vi "main.vi"() -> ()   [LabVIEW 2023] (continued)
"ScaleFac"=0.1, "ScaleOff"=0.0}, {"1802D0A6", "Frame"="INVTEACStat2\ndatabase", "NameShort"="INVTEACStat2OUTVolt", "StartBit"=16, "NumBits"=16, "Min"=0.0, "Max"=1000.0, "ScaleFac"=0.1, "ScaleOff"=0.0}, {"1801D0A5", "Frame"="INVTEHPSStat\ndatabase", "NameShort"="INVTEHPSFaultLvl", "StartBit"=8, "NumBits"=2, "Min"=0.0, "Max"=3.0, "ScaleFac"=1.0, "ScaleOff"=0.0}, {"1801D0A5", "Frame"="INVTEHPSStat\ndatabase", "NameShort"="INVTEHPSStatErrCode", "StartBit"=0, "NumBits"=8, "Min"=0.0, "Max"=255.0, "ScaleFac"=1.0, "ScaleOff"=0.0}, {"1801D0A5", "Frame"="INVTEHPSStat\ndatabase", "NameShort"="INVTEHPSStatFaultStat", "StartBit"=14, "NumBits"=2, "Min"=0.0, "Max"=3.0, "ScaleFac"=1.0, "ScaleOff"=0.0}, {"1801D0A5", "Frame"="INVTEHPSStat\ndatabase", "NameShort"="INVTEHPSStatINVolt", "StartBit"=16, "NumBits"=16, "Min"=0.0, "Max"=1000.0, "ScaleFac"=0.1, "ScaleOff"=0.0}, {"1801D0A5", "Frame"="INVTEHPSStat\ndatabase", "NameShort"="INVTEHPSStatInvertorTemp", "StartBit"=48, "NumBits"=8, "Min"=-40.0, "Max"=150.0, "ScaleFac"=1.0, "ScaleOff"=-40.0}, {"1801D0A5", "Frame"="INVTEHPSStat\ndatabase", "NameShort"="INVTEHPSStatLife", "StartBit"=56, "NumBits"=8, "Min"=0.0, "Max"=255.0, "ScaleFac"=1.0, "ScaleOff"=0.0}, {"1801D0A5", "Frame"="INVTEHPSStat\ndatabase", "NameShort"="INVTEHPSStatMtrTemp", "StartBit"=32, "NumBits"=8, "Min"=-40.0, "Max"=200.0, "ScaleFac"=1.0, "ScaleOff"=-40.0}, {"1801D0A5", "Frame"="INVTEHPSStat\ndatabase", "NameShort"="INVTEHPSStatPowerStat", "StartBit"=10, "NumBits"=2, "Min"=0.0, "Max"=3.0, "ScaleFac"=1.0, "ScaleOff"=0.0}, {"1801D0A5", "Frame"="INVTEHPSStat\ndatabase", "NameShort"="INVTEHPSStatWorkStat", "StartBit"=12, "NumBits"=2, "Min"=0.0, "Max"=3.0, "ScaleFac"=1.0, "ScaleOff"=0.0}, {"1802D0A5", "Frame"="INVTEHPSStat2\ndatabase", "NameShort"="INVTEHPSStat2INCurr", "StartBit"=48, "NumBits"=16, "Min"=0.0, "Max"=6553.5, "ScaleFac"=0.1, "ScaleOff"=0.0}, {"1802D0A5", "Frame"="INVTEHPSStat2\ndatabase", "NameShort"="INVTEHPSStat2Mtrrpm", "StartBit"=0, "NumBits"=16, "Min"=-5000.0, "Max"=5000.0, "ScaleFac"=0.5, "ScaleOff"=-5000.0}, {"1802D0A5", "Frame"="INVTEHPSStat2\ndatabase", "NameShort"="INVTEHPSStat2OUTCurr", "StartBit"=32, "NumBits"=16, "Min"=0.0, "Max"=500.0, "ScaleFac"=0.1, "ScaleOff"=0.0}, {"1802D0A5", "Frame"="INVTEHPSStat2\ndatabase", "NameShort"="INVTEHPSStat2OUTVolt", "StartBit"=16, "NumBits"=16, "Min"=0.0, "Max"=1000.0, "ScaleFac"=0.1, "ScaleOff"=0.0}, {"1801D0D7", "Frame"="INVTInsulationTester\ndatabase", "NameShort"="INVTInsulationTestErrorLv", "StartBit"=32, "NumBits"=8, "Min"=0.0, "Max"=255.0, "ScaleFac"=1.0, "ScaleOff"=0.0}, {"1801D0D7", "Frame"="INVTInsulationTester\ndatabase", "NameShort"="INVTInsulationTestLife", "StartBit"=40, "NumBits"=8, "Min"=0.0, "Max"=255.0, "ScaleFac"=1.0, "ScaleOff"=0.0}, {"1801D0D7", "Frame"="INVTInsulationTester\ndatabase", "NameShort"="INVTInsulationTestNEGtoGNDResist", "StartBit"=16, "NumBits"=16, "Min"=0.0, "Max"=65535.0, "ScaleFac"=1.0, "ScaleOff"=0.0}, {"1801D0D7", "Frame"="INVTInsulationTester\ndatabase", "NameShort"="INVTInsulationTestPOStoGNDResist", "StartBit"=0, "NumBits"=16, "Min"=0.0, "Max"=65535.0, "ScaleFac"=1.0, "ScaleOff"=0.0}, {"1801D0D7", "Frame"="INVTInsulationTester\ndatabase", "NameShort"="INVTInsulationTestStat", "StartBit"=48, "NumBits"=8, "Min"=0.0, "Max"=255.0, "ScaleFac"=1.0, "ScaleOff"=0.0}, {"18F301A8", "Frame"="INVTPDU\ndatabase", "NameShort"="INVTPDUACHVLoopStat", "StartBit"=26, "NumBits"=2, "Min"=0.0, "Max"=3.0, "ScaleFac"=1.0, "ScaleOff"=0.0}, {"18F301A8", "Frame"="INVTPDU\ndatabase", "NameShort"="INVTPDUACPrechrgRlyStat", "StartBit"=20, "NumBits"=2, "Min"=0.0, "Max"=3.0, "ScaleFac"=1.0, "ScaleOff"=0.0}, {"18F301A8", "Frame"="INVTPDU\ndatabase", "NameShort"="INVTPDUACRlyStat", "StartBit"=22, "NumBits"=2, "Min"=0.0, "Max"=3.0, "ScaleFac"=1.0, "ScaleOff"=0.0}, {"18F301A8", "Frame"="INVTPDU\ndatabase", "NameShort"="INVTPDUFaultLvl", "StartBit"=32, "NumBits"=2, "Min"=0.0, "Max"=3.0, "ScaleFac"=1.0, "ScaleOff"=0.0}, {"18F301A8", "Frame"="INVTPDU\ndatabase", "NameShort"="INVTPDULife", "StartBit"=56, "NumBits"=8, "Min"=0.0, "Max"=255.0, "ScaleFac"=1.0, "ScaleOff"=0.0}, {"18F301A8", "Frame"="INVTPDU\ndatabase", "NameShort"="INVTPDUMCUHVLoopStat", "StartBit"=2, "NumBits"=2, "Min"=0.0, "Max"=3.0, "ScaleFac"=1.0, "ScaleOff"=0.0}, {"18F301A8", "Frame"="INVTPDU\ndatabase", "NameShort"="INVTPDUMCUMainRlyStat", "StartBit"=4, "NumBits"=2, "Min"=0.0, "Max"=3.0, "ScaleFac"=1.0, "ScaleOff"=0.0}, {"18F301A8", "Frame"="INVTPDU\ndatabase", "NameShort"="INVTPDUMCUPrechrgRlyStat", "StartBit"=6, "NumBits"=2, "Min"=0.0, "Max"=3.0, "ScaleFac"=1.0, "ScaleOff"=0.0}, {"18F301A8", "Frame"="INVTPDU\ndatabase", "NameShort"="INVTPDUStat", "StartBit"=0, "NumBits"=2, "Min"=0.0, "Max"=3.0, "ScaleFac"=1.0, "ScaleOff"=0.0}, {"18F301B8", "Frame"="INVTPDU2\ndatabase", "NameShort"="INVTPDU2INVolt", "StartBit"=0, "NumBits"=16, "Min"=0.0, "Max"=6553.5, "ScaleFac"=0.1, "ScaleOff"=0.0}, {"18F43A17", "Frame"="IP\ndatabase", "NameShort"="IP24V", "StartBit"=0, "NumBits"=8, "Min"=0.0, "Max"=50.0, "ScaleFac"=0.2, "ScaleOff"=0.0}, {"18F43A17", "Frame"="IP\ndatabase", "NameShort"="IPACCKeyPosnStat", "StartBit"=15, "NumBits"=1, "Min"=0.0, "Max"=1.0, "ScaleFac"=1.0, "ScaleOff"=0.0}, {"18F43A17", "Frame"="IP\ndatabase", "NameShort"="IPFrontAirReservoirPressure", "StartBit"=16, "NumBits"=8, "Min"=0.0, "Max"=1.0, "ScaleFac"=0.01, "ScaleOff"=0.0}, {"18F43A17", "Frame"="IP\ndatabase", "NameShort"="IPFrontDoorStat", "StartBit"=10, "NumBits"=1, "Min"=0.0, "Max"=1.0, "ScaleFac"=1.0, "ScaleOff"=0.0}, {"18F43A17", "Frame"="IP\ndatabase", "NameShort"="IPHandbrkStat", "StartBit"=12, "NumBits"=1, "Min"=0.0, "Max"=1.0, "ScaleFac"=1.0, "ScaleOff"=0.0}, {"18F43A17", "Frame"="IP\ndatabase", "NameShort"="IPHatchDoorStat", "StartBit"=11, "NumBits"=1, "Min"=0.0, "Max"=1.0, "ScaleFac"=1.0, "ScaleOff"=0.0}, {"18F43A17", "Frame"="IP\ndatabase", "NameShort"="IPLife", "StartBit"=56, "NumBits"=8, "Min"=0.0, "Max"=255.0, "ScaleFac"=1.0, "ScaleOff"=0.0}, {"18F43A17", "Frame"="IP\ndatabase", "NameShort"="IPMidDoorStat", "StartBit"=9, "NumBits"=1, "Min"=0.0, "Max"=1.0, "ScaleFac"=1.0, "ScaleOff"=0.0}, {"18F43A17", "Frame"="IP\ndatabase", "NameShort"="IPONKeyPosnStat", "StartBit"=14, "NumBits"=1, "Min"=0.0, "Max"=1.0, "ScaleFac"=1.0, "ScaleOff"=0.0}, {"18F43A17", "Frame"="IP\ndatabase", "NameShort"="IPRearAirReservoirPressure", "StartBit"=24, "NumBits"=8, "Min"=0.0, "Max"=1.0, "ScaleFac"=0.01, "ScaleOff"=0.0}, {"18F43A17", "Frame"="IP\ndatabase", "NameShort"="IPRearDoorStat", "StartBit"=8, "NumBits"=1, "Min"=0.0, "Max"=1.0, "ScaleFac"=1.0, "ScaleOff"=0.0}, {"18F43A17", "Frame"="IP\ndatabase", "NameShort"="IPSmokeDetectStat", "StartBit"=13, "NumBits"=1, "Min"=0.0, "Max"=1.0, "ScaleFac"=1.0, "ScaleOff"=0.0}, {"18F43A17", "Frame"="IP\ndatabase", "NameShort"="IPSpeedLimitReq", "StartBit"=33, "NumBits"=1, "Min"=0.0, "Max"=1.0, "ScaleFac"=1.0, "ScaleOff"=0.0}, {"18F43A17", "Frame"="IP\ndatabase", "NameShort"="IPThrottleInterlockReq", "StartBit"=32, "NumBits"=1, "Min"=0.0, "Max"=1.0, "ScaleFac"=1.0, "ScaleOff"=0.0}, {"18A70017", "Frame"="IP2\ndatabase", "NameShort"="IP2ABSStat", "StartBit"=42, "NumBits"=2, "Min"=0.0, "Max"=3.0, "ScaleFac"=1.0, "ScaleOff"=0.0}, {"18A70017", "Frame"="IP2\ndatabase", "NameShort"="IP2AirConStat", "StartBit"=14, "NumBits"=2, "Min"=0.0, "Max"=3.0, "ScaleFac"=1.0, "ScaleOff"=0.0}, {"18A70017", "Frame"="IP2\ndatabase", "NameShort"="IP2AirFilterClogWarn", "StartBit"=10, "NumBits"=2, "Min"=0.0, "Max"=3.0, "ScaleFac"=1.0, "ScaleOff"=0.0}, {"18A70017", "Frame"="IP2\ndatabase", "NameShort"="IP2BrkPadsWornOutWarn", "StartBit"=8, "NumBits"=2, "Min"=0.0, "Max"=3.0, "ScaleFac"=1.0, "ScaleOff"=0.0}, {"18A70017", "Frame"="IP2\ndatabase", "NameShort"="IP2BrkPressureWarn", "StartBit"=2, "NumBits"=2, "Min"=0.0, "Max"=3.0, "ScaleFac"=1.0, "ScaleOff"=0.0}, {"18A70017", "Frame"="IP2\ndatabase", "NameShort"="IP2BrkStat", "StartBit"=36, "NumBits"=2, "Min"=0.0, "Max"=3.0, "ScaleFac"=1.0, "ScaleOff"=0.0}, {"18A70017", "Frame"="IP2\ndatabase", "NameShort"="IP2EHPSWarn", "StartBit"=4, "NumBits"=2, "Min"=0.0, "Max"=3.0, "ScaleFac"=1.0, "ScaleOff"=0.0}, {"18A70017", "Frame"="IP2\ndatabase", "NameShort"="IP2EngineOilTempWarn", "StartBit"=54, "NumBits"=2, "Min"=0.0, "Max"=3.0, "ScaleFac"=1.0, "ScaleOff"=0.0}, {"18A70017", "Frame"="IP2\ndatabase", "NameShort"="IP2FogLightSig", "StartBit"=26, "NumBits"=2, "Min"=0.0, "Max"=3.0, "ScaleFac"=1.0, "ScaleOff"=0.0}, {"18A70017", "Frame"="IP2\ndatabase", "NameShort"="IP2FrontDoorSig", "StartBit"=20, "NumBits"=2, "Min"=0.0, "Max"=3.0, "ScaleFac"=1.0, "ScaleOff"=0.0}, {"18A70017", "Frame"="IP2\ndatabase", "NameShort"="IP2FuelClogWarn", "StartBit"=52, "NumBits"=2, "Min"=0.0, "Max"=3.0, "ScaleFac"=1.0, "ScaleOff"=0.0}, {"18A70017", "Frame"="IP2\ndatabase", "NameShort"="IP2FuelGauge", "StartBit"=56, "NumBits"=8, "Min"=0.0, "Max"=100.0, "ScaleFac"=0.4, "ScaleOff"=0.0}, {"18A70017", "Frame"="IP2\ndatabase", "NameShort"="IP2FuelWarn", "StartBit"=12, "NumBits"=2, "Min"=0.0, "Max"=3.0, "ScaleFac"=1.0, "ScaleOff"=0.0}, {"18A70017", "Frame"="IP2\ndatabase", "NameShort"="IP2GearNSig", "StartBit"=16, "NumBits"=2, "Min"=0.0, "Max"=3.0, "ScaleFac"=1.0, "ScaleOff"=0.0}, {"18A70017", "Frame"="IP2\ndatabase", "NameShort"="IP2GearRSig", "StartBit"=18, "NumBits"=2, "Min"=0.0, "Max"=3.0, "ScaleFac"=1.0, "ScaleOff"=0.0}, {"18A70017", "Frame"="IP2\ndatabase", "NameShort"="IP2HandBrkStat", "StartBit"=38, "NumBits"=2, "Min"=0.0, "Max"=3.0, "ScaleFac"=1.0, "ScaleOff"=0.0}, {"18A70017", "Frame"="IP2\ndatabase", "NameShort"="IP2HeaterStat", "StartBit"=44, "NumBits"=2, "Min"=0.0, "Max"=3.0, "ScaleFac"=1.0, "ScaleOff"=0.0}, {"18A70017", "Frame"="IP2\ndatabase", "NameShort"="IP2HighBeamSig", "StartBit"=30, "NumBits"=2, "Min"=0.0, "Max"=3.0, "ScaleFac"=1.0, "ScaleOff"=0.0}, {"18A70017", "Frame"="IP2\ndatabase", "NameShort"="IP2HornSig", "StartBit"=24, "NumBits"=2, "Min"=0.0, "Max"=0.0, "ScaleFac"=1.0, "ScaleOff"=0.0}, {"18A70017", "Frame"="IP2\ndatabase", "NameShort"="IP2LeftTurnSig", "StartBit"=32, "NumBits"=2, "Min"=0.0, "Max"=3.0, "ScaleFac"=1.0, "ScaleOff"=0.0}, {"18A70017", "Frame"="IP2\ndatabase", "NameShort"="IP2LowBeamSig", "StartBit"=28, "NumBits"=2, "Min"=0.0, "Max"=3.0, "ScaleFac"=1.0, "ScaleOff"=0.0}, {"18A70017", "Frame"="IP2\ndatabase", "NameShort"="IP2LowWaterLvlWarn", "StartBit"=6, "NumBits"=2, "Min"=0.0, "Max"=3.0, "ScaleFac"=1.0, "ScaleOff"=0.0}, {"18A70017", "Frame"="IP2\ndatabase", "NameShort"="IP2MidDoorSig", "StartBit"=22, "NumBits"=2, "Min"=0.0, "Max"=3.0, "ScaleFac"=1.0, "ScaleOff"=0.0}, {"18A70017", "Frame"="IP2\ndatabase", "NameShort"="IP2OilFilterClogWarn", "StartBit"=50, "NumBits"=2, "Min"=0.0, "Max"=3.0, "ScaleFac"=1.0, "ScaleOff"=0.0}, {"18A70017", "Frame"="IP2\ndatabase", "NameShort"="IP2RegenLeverStat", "StartBit"=40, "NumBits"=2, "Min"=0.0, "Max"=3.0, "ScaleFac"=1.0, "ScaleOff"=0.0}, {"18A70017", "Frame"="IP2\ndatabase", "NameShort"="IP2RegenOverheatWarn", "StartBit"=46, "NumBits"=2, "Min"=0.0, "Max"=3.0, "ScaleFac"=1.0, "ScaleOff"=0.0}, {"18A70017", "Frame"="IP2\ndatabase", "NameShort"="IP2RightTurnSig", "StartBit"=34, "NumBits"=2, "Min"=0.0, "Max"=3.0, "ScaleFac"=1.0, "ScaleOff"=0.0}, {"18A70017", "Frame"="IP2\ndatabase", "NameShort"="IP2SmokeDetectorWarn", "StartBit"=48, "NumBits"=2, "Min"=0.0, "Max"=3.0, "ScaleFac"=1.0, "ScaleOff"=0.0}, {"18A70017", "Frame"="IP2\ndatabase", "NameShort"="IP2ThrottleInterlockWarn", "StartBit"=0, "NumBits"=2, "Min"=0.0, "Max"=3.0, "ScaleFac"=1.0, "ScaleOff"=0.0}, {"18FEC117", "Frame"="IPMileage\ndatabase", "NameShort"="IPMileageTotalOdometer", "StartBit"=0, "NumBits"=32, "Min"=0.0, "Max"=21055406.0, "ScaleFac"=0.005, "ScaleOff"=0.0}, {"18FEC117", "Frame"="IPMileage\ndatabase", "NameShort"="IPMileageTripA", "StartBit"=32, "NumBits"=32, "Min"=0.0, "Max"=21055406.0, "ScaleFac"=0.005, "ScaleOff"=0.0}, {"18F746E6", "Frame"="InsulationTesterS\ndatabase", "NameShort"="InsulatTesterSDetailedErrCode", "StartBit"=40, "NumBits"=8, "Min"=0.0, "Max"=255.0, "ScaleFac"=1.0, "ScaleOff"=0.0}, {"18F746E6", "Frame"="InsulationTesterS\ndatabase", "NameShort"="InsulatTesterSDeviceFailure", "StartBit"=53, "NumBits"=1, "Min"=0.0, "Max"=1.0, "ScaleFac"=1.0, "ScaleOff"=0.0}, {"18F746E6", "Frame"="InsulationTesterS\ndatabase", "NameShort"="InsulatTesterSHVLeakAlertLv", "StartBit"=0, "NumBits"=3, "Min"=0.0, "Max"=7.0, "ScaleFac"=1.0, "ScaleOff"=0.0}, {"18F746E6", "Frame"="InsulationTesterS\ndatabase", "NameShort"="InsulatTesterSHVNegInsultErr", "StartBit"=51, "NumBits"=1, "Min"=0.0, "Max"=1.0, "ScaleFac"=1.0, "ScaleOff"=0.0}, {"18F746E6", "Frame"="InsulationTesterS\ndatabase", "NameShort"="InsulatTesterSHVPosInsltErr", "StartBit"=50, "NumBits"=1, "Min"=0.0, "Max"=1.0, "ScaleFac"=1.0, "ScaleOff"=0.0}, {"18F746E6", "Frame"="InsulationTesterS\ndatabase", "NameShort"="InsulatTesterSLife", "StartBit"=56, "NumBits"=8, "Min"=0.0, "Max"=255.0, "ScaleFac"=1.0, "ScaleOff"=0.0}, {"18F746E6", "Frame"="InsulationTesterS\ndatabase", "NameShort"="InsulatTesterSLv1Alert", "StartBit"=48, "NumBits"=1, "Min"=0.0, "Max"=1.0, "ScaleFac"=1.0, "ScaleOff"=0.0}, {"18F746E6", "Frame"="InsulationTesterS\ndatabase", "NameShort"="InsulatTesterSLv2Alert", "StartBit"=49, "NumBits"=1, "Min"=0.0, "Max"=1.0, "ScaleFac"=1.0, "ScaleOff"=0.0}, {"18F746E6", "Frame"="InsulationTesterS\ndatabase", "NameShort"="InsulatTesterSNegInsulatResist", "StartBit"=24, "NumBits"=16, "Min"=0.0, "Max"=65535.0, "ScaleFac"=1.0, "ScaleOff"=0.0}, {"18F746E6", "Frame"="InsulationTesterS\ndatabase", "NameShort"="InsulatTesterSPosInsulatResist", "StartBit"=8, "NumBits"=16, "Min"=0.0, "Max"=65535.0, "ScaleFac"=1.0, "ScaleOff"=0.0}, {"18F746E6", "Frame"="InsulationTesterS\ndatabase", "NameShort"="InsulatTesterSWiringFailure", "StartBit"=52, "NumBits"=1, "Min"=0.0, "Max"=1.0, "ScaleFac"=1.0, "ScaleOff"=0.0}, {"18F11FF0", "Frame"="MCU1ElectricalStat\ndatabase", "NameShort"="MCU1CANBusConnectStat", "StartBit"=52, "NumBits"=1, "Min"=0.0, "Max"=1.0, "ScaleFac"=1.0, "ScaleOff"=0.0}, {"18F11FF0", "Frame"="MCU1ElectricalStat\ndatabase", "NameShort"="MCU1HPINCurr", "StartBit"=16, "NumBits"=16, "Min"=-1000.0, "Max"=1000.0, "ScaleFac"=0.1, "ScaleOff"=-1000.0}, {"18F11FF0", "Frame"="MCU1ElectricalStat\ndatabase", "NameShort"="MCU1HPINOvercurrErr", "StartBit"=43, "NumBits"=1, "Min"=0.0, "Max"=1.0, "ScaleFac"=1.0, "ScaleOff"=0.0}, {"18F11FF0", "Frame"="MCU1ElectricalStat\ndatabase", "NameShort"="MCU1HPINOvervoltErr", "StartBit"=40, "NumBits"=1, "Min"=0.0, "Max"=1.0, "ScaleFac"=1.0, "ScaleOff"=0.0}, {"18F11FF0", "Frame"="MCU1ElectricalStat\ndatabase", "NameShort"="MCU1HPINUndervoltErr", "StartBit"=44, "NumBits"=1, "Min"=0.0, "Max"=1.0, "ScaleFac"=1.0, "ScaleOff"=0.0}, {"18F11FF0", "Frame"="MCU1ElectricalStat\ndatabase", "NameShort"="MCU1HPINVolt", "StartBit"=0, "NumBits"=16, "Min"=0.0, "Max"=1000.0, "ScaleFac"=0.1, "ScaleOff"=0.0}, {"18F11FF0", "Frame"="MCU1ElectricalStat\ndatabase", "NameShort"="MCU1HVBattConnectStat", "StartBit"=55, "NumBits"=1, "Min"=0.0, "Max"=1.0, "ScaleFac"=1.0, "ScaleOff"=0.0}, {"18F11FF0", "Frame"="MCU1ElectricalStat\ndatabase", "NameShort"="MCU1HillStartStat", "StartBit"=39, "NumBits"=1, "Min"=0.0, "Max"=1.0, "ScaleFac"=1.0, "ScaleOff"=0.0}, {"18F11FF0", "Frame"="MCU1ElectricalStat\ndatabase", "NameShort"="MCU1KeyIgniteStat", "StartBit"=54, "NumBits"=1, "Min"=0.0, "Max"=1.0, "ScaleFac"=1.0, "ScaleOff"=0.0}, {"18F11FF0", "Frame"="MCU1ElectricalStat\ndatabase", "NameShort"="MCU1LVDCPowErr", "StartBit"=53, "NumBits"=1, "Min"=0.0, "Max"=1.0, "ScaleFac"=1.0, "ScaleOff"=0.0}, {"18F11FF0", "Frame"="MCU1ElectricalStat\ndatabase", "NameShort"="MCU1Life", "StartBit"=60, "NumBits"=4, "Min"=0.0, "Max"=15.0, "ScaleFac"=1.0, "ScaleOff"=0.0}, {"18F11FF0", "Frame"="MCU1ElectricalStat\ndatabase", "NameShort"="MCU1MCUErr", "StartBit"=33, "NumBits"=1, "Min"=0.0, "Max"=1.0, "ScaleFac"=1.0, "ScaleOff"=0.0}, {"18F11FF0", "Frame"="MCU1ElectricalStat\ndatabase", "NameShort"="MCU1McuOverheatErr", "StartBit"=46, "NumBits"=1, "Min"=0.0, "Max"=1.0, "ScaleFac"=1.0, "ScaleOff"=0.0}, {"18F11FF0", "Frame"="MCU1ElectricalStat\ndatabase", "NameShort"="MCU1McuTempAlert", "StartBit"=51, "NumBits"=1, "Min"=0.0, "Max"=1.0, "ScaleFac"=1.0, "ScaleOff"=0.0}, {"18F11FF0", "Frame"="MCU1ElectricalStat\ndatabase", "NameShort"="MCU1Mode", "StartBit"=34, "NumBits"=5, "Min"=0.0, "Max"=31.0, "ScaleFac"=1.0, "ScaleOff"=0.0}, {"18F11FF0", "Frame"="MCU1ElectricalStat\ndatabase", "NameShort"="MCU1MtrOverheatErr", "StartBit"=45, "NumBits"=1, "Min"=0.0, "Max"=1.0, "ScaleFac"=1.0, "ScaleOff"=0.0}, {"18F11FF0", "Frame"="MCU1ElectricalStat\ndatabase", "NameShort"="MCU1MtrOverspdErr", "StartBit"=47, "NumBits"=1, "Min"=0.0, "Max"=1.0, "ScaleFac"=1.0, "ScaleOff"=0.0}, {"18F11FF0", "Frame"="MCU1ElectricalStat\ndatabase", "NameShort"="MCU1MtrPosnSensorErr", "StartBit"=42, "NumBits"=1, "Min"=0.0, "Max"=1.0, "ScaleFac"=1.0, "ScaleOff"=0.0}, {"18F11FF0", "Frame"="MCU1ElectricalStat\ndatabase", "NameShort"="MCU1MtrTempAlert", "StartBit"=50, "NumBits"=1, "Min"=0.0, "Max"=1.0, "ScaleFac"=1.0, "ScaleOff"=0.0}, {"18F11FF0", "Frame"="MCU1ElectricalStat\ndatabase", "NameShort"="MCU1NoPermsToOp", "StartBit"=57, "NumBits"=1, "Min"=0.0, "Max"=1.0, "ScaleFac"=1.0, "ScaleOff"=0.0}, {"18F11FF0", "Frame"="MCU1ElectricalStat\ndatabase", "NameShort"="MCU1PermsToOp", "StartBit"=56, "NumBits"=1, "Min"=0.0, "Max"=1.0, "ScaleFac"=1.0, "ScaleOff"=0.0}, {"18F11FF0", "Frame"="MCU1ElectricalStat\ndatabase", "NameShort"="MCU1PhaseCurrErr", "StartBit"=32, "NumBits"=1, "Min"=0.0, "Max"=1.0, "ScaleFac"=1.0, "ScaleOff"=0.0}, {"18F11FF0", "Frame"="MCU1ElectricalStat\ndatabase", "NameShort"="MCU1PhaseUOvercurrErr", "StartBit"=48, "NumBits"=1, "Min"=0.0, "Max"=1.0, "ScaleFac"=1.0, "ScaleOff"=0.0}, {"18F11FF0", "Frame"="MCU1ElectricalStat\ndatabase", "NameShort"="MCU1PhaseWOvercurrErr", "StartBit"=49, "NumBits"=1, "Min"=0.0, "Max"=1.0, "ScaleFac"=1.0, "ScaleOff"=0.0}, {"18F120F0", "Frame"="MCU2MtrStat\ndatabase", "NameShort"="MCU2CurrentMtrRPM", "StartBit"=16, "NumBits"=16, "Min"=-12000.0, "Max"=12000.0, "ScaleFac"=1.0, "ScaleOff"=-12000.0}, {"18F120F0", "Frame"="MCU2MtrStat\ndatabase", "NameShort"="MCU2McuTemp", "StartBit"=56, "NumBits"=8, "Min"=-40.0, "Max"=210.0, "ScaleFac"=1.0, "ScaleOff"=-40.0}, {"18F120F0", "Frame"="MCU2MtrStat\ndatabase", "NameShort"="MCU2MtrActualTorq", "StartBit"=32, "NumBits"=16, "Min"=-3000.0, "Max"=3000.0, "ScaleFac"=0.1, "ScaleOff"=-3000.0}, {"18F120F0", "Frame"="MCU2MtrStat\ndatabase", "NameShort"="MCU2MtrPeakTorq", "StartBit"=0, "NumBits"=16, "Min"=-3000.0, "Max"=3000.0, "ScaleFac"=0.1, "ScaleOff"=-3000.0}, {"18F120F0", "Frame"="MCU2MtrStat\ndatabase", "NameShort"="MCU2MtrTemp", "StartBit"=48, "NumBits"=8, "Min"=-40.0, "Max"=210.0, "ScaleFac"=1.0, "ScaleOff"=-40.0}, {"18F121F0", "Frame"="MCU3ErrorStat\ndatabase", "NameShort"="MCU3DriveshaftTorq", "StartBit"=48, "NumBits"=16, "Min"=-3000.0, "Max"=3000.0, "ScaleFac"=0.1, "ScaleOff"=-3000.0}, {"18F121F0", "Frame"="MCU3ErrorStat\ndatabase", "NameShort"="MCU3ErrCode", "StartBit"=8, "NumBits"=8, "Min"=0.0, "Max"=255.0, "ScaleFac"=1.0, "ScaleOff"=0.0}, {"18F121F0", "Frame"="MCU3ErrorStat\ndatabase", "NameShort"="MCU3ErrLv", "StartBit"=4, "NumBits"=4, "Min"=0.0, "Max"=4.0, "ScaleFac"=1.0, "ScaleOff"=0.0}, {"18F121F0", "Frame"="MCU3ErrorStat\ndatabase", "NameShort"="MCU3HwVer", "StartBit"=27, "NumBits"=5, "Min"=0.0, "Max"=31.0, "ScaleFac"=1.0, "ScaleOff"=0.0}, {"18F121F0", "Frame"="MCU3ErrorStat\ndatabase", "NameShort"="MCU3SwVer", "StartBit"=16, "NumBits"=11, "Min"=0.0, "Max"=2047.0, "ScaleFac"=1.0, "ScaleOff"=0.0}, {"18F121F0", "Frame"="MCU3ErrorStat\ndatabase", "NameShort"="MCU3SysStat", "StartBit"=0, "NumBits"=4, "Min"=0.0, "Max"=6.0, "ScaleFac"=1.0, "ScaleOff"=0.0}, {"1FFFFFFC", "Frame"="PCINPUT\ndatabase", "NameShort"="PCRXMsg1", "StartBit"=0, "NumBits"=16, "Min"=0.0, "Max"=65.535, "ScaleFac"=0.001, "ScaleOff"=0.0}, {"1FFFFFFC", "Frame"="PCINPUT\ndatabase", "NameShort"="PCRXMsg3", "StartBit"=16, "NumBits"=16, "Min"=0.0, "Max"=65.535, "ScaleFac"=0.001, "ScaleOff"=0.0}, {"1FFFFFFC", "Frame"="PCINPUT\ndatabase", "NameShort"="PCRXMsg5", "StartBit"=32, "NumBits"=16, "Min"=0.0, "Max"=65.535, "ScaleFac"=0.001, "ScaleOff"=0.0}, {"1FFFFFFC", "Frame"="PCINPUT\ndatabase", "NameShort"="PCRXMsg7", "StartBit"=48, "NumBits"=16, "Min"=0.0, "Max"=65.535, "ScaleFac"=0.001, "ScaleOff"=0.0}, {"1FFFFFFD", "Frame"="PCOUTPUT\ndatabase", "NameShort"="PCTXMsg1", "StartBit"=0, "NumBits"=16, "Min"=0.0, "Max"=65.535, "ScaleFac"=0.001, "ScaleOff"=0.0}, {"1FFFFFFD", "Frame"="PCOUTPUT\ndatabase", "NameShort"="PCTXMsg3", "StartBit"=16, "NumBits"=16, "Min"=0.0, "Max"=65.535, "ScaleFac"=0.001, "ScaleOff"=0.0}, {"1FFFFFFD", "Frame"="PCOUTPUT\ndatabase", "NameShort"="PCTXMsg5", "StartBit"=32, "NumBits"=16, "Min"=0.0, "Max"=65.535, "ScaleFac"=0.001, "ScaleOff"=0.0}, {"1FFFFFFD", "Frame"="PCOUTPUT\ndatabase", "NameShort"="PCTXMsg7", "StartBit"=48, "NumBits"=16, "Min"=0.0, "Max"=65.535, "ScaleFac"=0.001, "ScaleOff"=0.0}, {"1FFFFFFE", "Frame"="PCRX\ndatabase", "NameShort"="PCRXMsg1", "StartBit"=0, "NumBits"=8, "Min"=0.0, "Max"=255.0, "ScaleFac"=1.0, "ScaleOff"=0.0}, {"1FFFFFFE", "Frame"="PCRX\ndatabase", "NameShort"="PCRXMsg2", "StartBit"=8, "NumBits"=8, "Min"=0.0, "Max"=255.0, "ScaleFac"=1.0, "ScaleOff"=0.0}, {"1FFFFFFE", "Frame"="PCRX\ndatabase", "NameShort"="PCRXMsg3", "StartBit"=16, "NumBits"=8, "Min"=0.0, "Max"=255.0, "ScaleFac"=1.0, "ScaleOff"=0.0}, {"1FFFFFFE", "Frame"="PCRX\ndatabase", "NameShort"="PCRXMsg4", "StartBit"=24, "NumBits"=8, "Min"=0.0, "Max"=255.0, "ScaleFac"=1.0, "ScaleOff"=0.0}, {"1FFFFFFE", "Frame"="PCRX\ndatabase", "NameShort"="PCRXMsg5", "StartBit"=32, "NumBits"=8, "Min"=0.0, "Max"=255.0, "ScaleFac"=1.0, "ScaleOff"=0.0}, {"1FFFFFFE", "Frame"="PCRX\ndatabase", "NameShort"="PCRXMsg6", "StartBit"=40, "NumBits"=8, "Min"=0.0, "Max"=255.0, "ScaleFac"=1.0, "ScaleOff"=0.0}, {"1FFFFFFE", "Frame"="PCRX\ndatabase", "NameShort"="PCRXMsg7", "StartBit"=48, "NumBits"=8, "Min"=0.0, "Max"=255.0, "ScaleFac"=1.0, "ScaleOff"=0.0}, {"1FFFFFFE", "Frame"="PCRX\ndatabase", "NameShort"="PCRXMsg8", "StartBit"=56, "NumBits"=8, "Min"=0.0, "Max"=255.0, "ScaleFac"=1.0, "ScaleOff"=0.0}, {"1FFFFFFF", "Frame"="PCTX\ndatabase", "NameShort"="PCTXMSDI_Gear", "StartBit"=0, "NumBits"=8, "Min"=0.0, "Max"=255.0, "ScaleFac"=1.0, "ScaleOff"=0.0}, {"1FFFFFFF", "Frame"="PCTX\ndatabase", "NameShort"="PCTXMsg2", "StartBit"=8, "NumBits"=8, "Min"=0.0, "Max"=255.0, "ScaleFac"=1.0, "ScaleOff"=0.0}, {"1FFFFFFF", "Frame"="PCTX\ndatabase", "NameShort"="PCTXMsg3", "StartBit"=16, "NumBits"=8, "Min"=0.0, "Max"=255.0, "ScaleFac"=1.0, "ScaleOff"=0.0}, {"1FFFFFFF", "Frame"="PCTX\ndatabase", "NameShort"="PCTXMsg4", "StartBit"=24, "NumBits"=8, "Min"=0.0, "Max"=255.0, "ScaleFac"=1.0, "ScaleOff"=0.0}, {"1FFFFFFF", "Frame"="PCTX\ndatabase", "NameShort"="PCTXMsg5", "StartBit"=32, "NumBits"=8, "Min"=0.0, "Max"=255.0, "ScaleFac"=1.0, "ScaleOff"=0.0}, {"1FFFFFFF", "Frame"="PCTX\ndatabase", "NameShort"="PCTXMsg6", "StartBit"=40, "NumBits"=8, "Min"=0.0, "Max"=255.0, "ScaleFac"=1.0, "ScaleOff"=0.0}, {"1FFFFFFF", "Frame"="PCTX\ndatabase", "NameShort"="PCTXMsg7", "StartBit"=48, "NumBits"=8, "Min"=0.0, "Max"=255.0, "ScaleFac"=1.0, "ScaleOff"=0.0}, {"1FFFFFFF", "Frame"="PCTX\ndatabase", "NameShort"="PCTXMsg8", "StartBit"=56, "NumBits"=8, "Min"=0.0, "Max"=255.0, "ScaleFac"=1.0, "ScaleOff"=0.0}, {"1828A796", "Frame"="SmokeDetector\ndatabase", "NameShort"="SmokeDetectorAlertDeviceAlert", "StartBit"=52, "NumBits"=2, "Min"=0.0, "Max"=1.0, "ScaleFac"=1.0, "ScaleOff"=0.0}, {"1828A796", "Frame"="SmokeDetector\ndatabase", "NameShort"="SmokeDetectorAlertSmokeAlert", "StartBit"=48, "NumBits"=2, "Min"=0.0, "Max"=1.0, "ScaleFac"=1.0, "ScaleOff"=0.0}, {"1828A796", "Frame"="SmokeDetector\ndatabase", "NameShort"="SmokeDetectorAlertTempAlert", "StartBit"=50, "NumBits"=2, "Min"=0.0, "Max"=1.0, "ScaleFac"=1.0, "ScaleOff"=0.0}, {"1828A796", "Frame"="SmokeDetector\ndatabase", "NameShort"="SmokeDetectorLife", "StartBit"=56, "NumBits"=8, "Min"=0.0, "Max"=255.0, "ScaleFac"=1.0, "ScaleOff"=0.0}, {"CF101A7", "Frame"="VCU01toIP\ndatabase", "NameShort"="VCU01BrkPedalDepth", "StartBit"=32, "NumBits"=8, "Min"=0.0, "Max"=100.0, "ScaleFac"=0.4, "ScaleOff"=0.0}, {"CF101A7", "Frame"="VCU01toIP\ndatabase", "NameShort"="VCU01BrkPedalStat", "StartBit"=7, "NumBits"=1, "Min"=0.0, "Max"=1.0, "ScaleFac"=1.0, "ScaleOff"=0.0}, {"CF101A7", "Frame"="VCU01toIP\ndatabase", "NameShort"="VCU01CarSpeed", "StartBit"=16, "NumBits"=16, "Min"=0.0, "Max"=200.0, "ScaleFac"=0.00390625, "ScaleOff"=0.0}, {"CF101A7", "Frame"="VCU01toIP\ndatabase", "NameShort"="VCU01DrivingMode", "StartBit"=0, "NumBits"=2, "Min"=0.0, "Max"=3.0, "ScaleFac"=1.0, "ScaleOff"=0.0}, {"CF101A7", "Frame"="VCU01toIP\ndatabase", "NameShort"="VCU01EESysMalfuctStat", "StartBit"=54, "NumBits"=1, "Min"=0.0, "Max"=1.0, "ScaleFac"=1.0, "ScaleOff"=0.0}, {"CF101A7", "Frame"="VCU01toIP\ndatabase", "NameShort"="VCU01ErrCode", "StartBit"=40, "NumBits"=8, "Min"=0.0, "Max"=255.0, "ScaleFac"=1.0, "ScaleOff"=0.0}, {"CF101A7", "Frame"="VCU01toIP\ndatabase", "NameShort"="VCU01GasPedalDepth", "StartBit"=8, "NumBits"=8, "Min"=0.0, "Max"=100.0, "ScaleFac"=0.4, "ScaleOff"=0.0}, {"CF101A7", "Frame"="VCU01toIP\ndatabase", "NameShort"="VCU01GearStat", "StartBit"=2, "NumBits"=4, "Min"=0.0, "Max"=15.0, "ScaleFac"=1.0, "ScaleOff"=0.0}, {"CF101A7", "Frame"="VCU01toIP\ndatabase", "NameShort"="VCU01HandBrkStat", "StartBit"=6, "NumBits"=1, "Min"=0.0, "Max"=1.0, "ScaleFac"=1.0, "ScaleOff"=0.0}, {"CF101A7", "Frame"="VCU01toIP\ndatabase", "NameShort"="VCU01HillstartAssistIconStat", "StartBit"=50, "NumBits"=1, "Min"=0.0, "Max"=1.0, "ScaleFac"=1.0, "ScaleOff"=0.0}, {"CF101A7", "Frame"="VCU01toIP\ndatabase", "NameShort"="VCU01Life", "StartBit"=56, "NumBits"=8, "Min"=0.0, "Max"=255.0, "ScaleFac"=1.0, "ScaleOff"=0.0}, {"CF101A7", "Frame"="VCU01toIP\ndatabase", "NameShort"="VCU01PowLimitedStat", "StartBit"=49, "NumBits"=1, "Min"=0.0, "Max"=1.0, "ScaleFac"=1.0, "ScaleOff"=0.0}, {"CF101A7", "Frame"="VCU01toIP\ndatabase", "NameShort"="VCU01SysReadyStat", "StartBit"=55, "NumBits"=1, "Min"=0.0, "Max"=1.0, "ScaleFac"=1.0, "ScaleOff"=0.0}, {"CF102A7", "Frame"="VCU02MtrNBMSRelayStat\ndatabase", "NameShort"="VCU02BattOpMode", "StartBit"=38, "NumBits"=2, "Min"=0.0, "Max"=3.0, "ScaleFac"=1.0, "ScaleOff"=0.0}, {"CF102A7", "Frame"="VCU02MtrNBMSRelayStat\ndatabase", "NameShort"="VCU02MtrEnblStat", "StartBit"=37, "NumBits"=1, "Min"=0.0, "Max"=1.0, "ScaleFac"=1.0, "ScaleOff"=0.0}, {"CF102A7", "Frame"="VCU02MtrNBMSRelayStat\ndatabase", "NameShort"="VCU02MtrOpMode", "StartBit"=32, "NumBits"=5, "Min"=0.0, "Max"=31.0, "ScaleFac"=1.0, "ScaleOff"=0.0}, {"CF102A7", "Frame"="VCU02MtrNBMSRelayStat\ndatabase", "NameShort"="VCU02MtrTargetSpeed", "StartBit"=16, "NumBits"=16, "Min"=-12000.0, "Max"=12000.0, "ScaleFac"=1.0, "ScaleOff"=-12000.0}, {"CF102A7", "Frame"="VCU02MtrNBMSRelayStat\ndatabase", "NameShort"="VCU02MtrTargetTorq", "StartBit"=0, "NumBits"=16, "Min"=0.0, "Max"=4095.0, "ScaleFac"=1.0, "ScaleOff"=0.0}, {"CF102A7", "Frame"="VCU02MtrNBMSRelayStat\ndatabase", "NameShort"="VCU02NegRelayStat", "StartBit"=59, "NumBits"=1, "Min"=0.0, "Max"=1.0, "ScaleFac"=1.0, "ScaleOff"=0.0}, {"CF102A7", "Frame"="VCU02MtrNBMSRelayStat\ndatabase", "NameShort"="VCU02PosRelayStat", "StartBit"=58, "NumBits"=1, "Min"=0.0, "Max"=1.0, "ScaleFac"=1.0, "ScaleOff"=0.0}, {"CF102A7", "Frame"="VCU02MtrNBMSRelayStat\ndatabase", "NameShort"="VCU02PrechgRelayStat", "StartBit"=57, "NumBits"=1, "Min"=0.0, "Max"=1.0, "ScaleFac"=1.0, "ScaleOff"=0.0}, {"CF103A7", "Frame"="VCU03VerNFiveInOneRelayStat\ndatabase", "NameShort"="VCU03AirComprNDCDCNEhpsRelayStat", "StartBit"=51, "NumBits"=1, "Min"=0.0, "Max"=1.0, "ScaleFac"=1.0, "ScaleOff"=0.0}, {"CF103A7", "Frame"="VCU03VerNFiveInOneRelayStat\ndatabase", "NameShort"="VCU03AirConRelayStat", "StartBit"=52, "NumBits"=1, "Min"=0.0, "Max"=1.0, "ScaleFac"=1.0, "ScaleOff"=0.0}, {"CF103A7", "Frame"="VCU03VerNFiveInOneRelayStat\ndatabase", "NameShort"="VCU03BattChgRelayCmd", "StartBit"=54, "NumBits"=1, "Min"=0.0, "Max"=1.0, "ScaleFac"=1.0, "ScaleOff"=0.0}, {"CF103A7", "Frame"="VCU03VerNFiveInOneRelayStat\ndatabase", "NameShort"="VCU03BattMainRelayCmd", "StartBit"=55, "NumBits"=1, "Min"=0.0, "Max"=1.0, "ScaleFac"=1.0, "ScaleOff"=0.0}, {"CF103A7", "Frame"="VCU03VerNFiveInOneRelayStat\ndatabase", "NameShort"="VCU03BowtypeChgCmd", "StartBit"=47, "NumBits"=1, "Min"=0.0, "Max"=1.0, "ScaleFac"=1.0, "ScaleOff"=0.0}, {"CF103A7", "Frame"="VCU03VerNFiveInOneRelayStat\ndatabase", "NameShort"="VCU03CompanyCode", "StartBit"=0, "NumBits"=8, "Min"=0.0, "Max"=255.0, "ScaleFac"=1.0, "ScaleOff"=0.0}, {"CF103A7", "Frame"="VCU03VerNFiveInOneRelayStat\ndatabase", "NameShort"="VCU03DefrostRelayStat", "StartBit"=53, "NumBits"=1, "Min"=0.0, "Max"=1.0, "ScaleFac"=1.0, "ScaleOff"=0.0}, {"CF103A7", "Frame"="VCU03VerNFiveInOneRelayStat\ndatabase", "NameShort"="VCU03DriveShaftSpeed", "StartBit"=24, "NumBits"=16, "Min"=-12000.0, "Max"=12000.0, "ScaleFac"=1.0, "ScaleOff"=-12000.0}, {"CF103A7", "Frame"="VCU03VerNFiveInOneRelayStat\ndatabase", "NameShort"="VCU03HVEmergCutoff", "StartBit"=48, "NumBits"=1, "Min"=0.0, "Max"=1.0, "ScaleFac"=1.0, "ScaleOff"=0.0}, {"CF103A7", "Frame"="VCU03VerNFiveInOneRelayStat\ndatabase", "NameShort"="VCU03HwVer", "StartBit"=19, "NumBits"=5, "Min"=0.0, "Max"=31.0, "ScaleFac"=1.0, "ScaleOff"=0.0}, {"CF103A7", "Frame"="VCU03VerNFiveInOneRelayStat\ndatabase", "NameShort"="VCU03Life", "StartBit"=56, "NumBits"=8, "Min"=0.0, "Max"=255.0, "ScaleFac"=1.0, "ScaleOff"=0.0}, {"CF103A7", "Frame"="VCU03VerNFiveInOneRelayStat\ndatabase", "NameShort"="VCU03MtrRelayStat", "StartBit"=50, "NumBits"=1, "Min"=0.0, "Max"=1.0, "ScaleFac"=1.0, "ScaleOff"=0.0}, {"CF103A7", "Frame"="VCU03VerNFiveInOneRelayStat\ndatabase", "NameShort"="VCU03PantographStat", "StartBit"=45, "NumBits"=2, "Min"=0.0, "Max"=3.0, "ScaleFac"=1.0, "ScaleOff"=0.0}, {"CF103A7", "Frame"="VCU03VerNFiveInOneRelayStat\ndatabase", "NameShort"="VCU03PrechgRelayStat", "StartBit"=49, "NumBits"=1, "Min"=0.0, "Max"=1.0, "ScaleFac"=1.0, "ScaleOff"=0.0}, {"CF103A7", "Frame"="VCU03VerNFiveInOneRelayStat\ndatabase", "NameShort"="VCU03SwVer", "StartBit"=8, "NumBits"=11, "Min"=0.0, "Max"=2047.0, "ScaleFac"=1.0, "ScaleOff"=0.0}, {"CF104A7", "Frame"="VCU04toEHPS\ndatabase", "NameShort"="VCU04EHPSAssignRPM", "StartBit"=8, "NumBits"=16, "Min"=0.0, "Max"=5000.0, "ScaleFac"=0.125, "ScaleOff"=0.0}, {"CF104A7", "Frame"="VCU04toEHPS\ndatabase", "NameShort"="VCU04EHPSEnbl1", "StartBit"=0, "NumBits"=2, "Min"=0.0, "Max"=3.0, "ScaleFac"=1.0, "ScaleOff"=0.0}, {"CF104A7", "Frame"="VCU04toEHPS\ndatabase", "NameShort"="VCU04EHPSEnbl2", "StartBit"=2, "NumBits"=2, "Min"=0.0, "Max"=3.0, "ScaleFac"=1.0, "ScaleOff"=0.0}, {"CF104A7", "Frame"="VCU04toEHPS\ndatabase", "NameShort"="VCU04EHPSLVEnbl", "StartBit"=24, "NumBits"=2, "Min"=0.0, "Max"=3.0, "ScaleFac"=1.0, "ScaleOff"=0.0}, {"CF104A7", "Frame"="VCU04toEHPS\ndatabase", "NameShort"="VCU04EHPSLife", "StartBit"=56, "NumBits"=8, "Min"=0.0, "Max"=255.0, "ScaleFac"=1.0, "ScaleOff"=0.0}, {"C3C4D4A", "Frame"="VCU05toAirCon\ndatabase", "NameShort"="VCU05AirConEnbl", "StartBit"=6, "NumBits"=1, "Min"=0.0, "Max"=1.0, "ScaleFac"=1.0, "ScaleOff"=0.0}, {"C3C4D4A", "Frame"="VCU05toAirCon\ndatabase", "NameShort"="VCU05AirConLife", "StartBit"=56, "NumBits"=8, "Min"=0.0, "Max"=255.0, "ScaleFac"=1.0, "ScaleOff"=0.0}, {"C3C4D4A", "Frame"="VCU05toAirCon\ndatabase", "NameShort"="VCU05AirConRead24VVolt", "StartBit"=32, "NumBits"=8, "Min"=0.0, "Max"=40.0, "ScaleFac"=1.0, "ScaleOff"=0.0}, {"C3C4D4A", "Frame"="VCU05toAirCon\ndatabase", "NameShort"="VCU05AirConReadSOC", "StartBit"=48, "NumBits"=16, "Min"=0.0, "Max"=100.0, "ScaleFac"=0.4, "ScaleOff"=0.0}, {"C3C4D4A", "Frame"="VCU05toAirCon\ndatabase", "NameShort"="VCU05AirConResetCmd", "StartBit"=0, "NumBits"=1, "Min"=0.0, "Max"=1.0, "ScaleFac"=1.0, "ScaleOff"=0.0}, {"C3C4D4A", "Frame"="VCU05toAirCon\ndatabase", "NameShort"="VCU05AirConRsvdUsing1", "StartBit"=31, "NumBits"=1, "Min"=0.0, "Max"=1.0, "ScaleFac"=1.0, "ScaleOff"=0.0}, {"CF105A7", "Frame"="VCU06toDCDC\ndatabase", "NameShort"="VCU06DCDCEnblCmd", "StartBit"=24, "NumBits"=8, "Min"=0.0, "Max"=255.0, "ScaleFac"=1.0, "ScaleOff"=0.0}, {"CF105A7", "Frame"="VCU06toDCDC\ndatabase", "NameShort"="VCU06DCDCEnblReqOutOf24V", "StartBit"=16, "NumBits"=8, "Min"=0.0, "Max"=255.0, "ScaleFac"=1.0, "ScaleOff"=0.0}, {"CF105A7", "Frame"="VCU06toDCDC\ndatabase", "NameShort"="VCU06DCDCLife", "StartBit"=56, "NumBits"=8, "Min"=0.0, "Max"=255.0, "ScaleFac"=1.0, "ScaleOff"=0.0}, {"CF105A7", "Frame"="VCU06toDCDC\ndatabase", "NameShort"="VCU06DCDCMinHVReq", "StartBit"=0, "NumBits"=16, "Min"=0.0, "Max"=6553.5, "ScaleFac"=0.1, "ScaleOff"=0.0}, {"18F106A7", "Frame"="VCU07toFiveInOneRelay\ndatabase", "NameShort"="VCU07FiveInOneAirComprRelayCmd", "StartBit"=3, "NumBits"=1, "Min"=0.0, "Max"=1.0, "ScaleFac"=1.0, "ScaleOff"=0.0}, {"18F106A7", "Frame"="VCU07toFiveInOneRelay\ndatabase", "NameShort"="VCU07FiveInOneAirConRelayCmd", "StartBit"=2, "NumBits"=1, "Min"=0.0, "Max"=1.0, "ScaleFac"=1.0, "ScaleOff"=0.0}, {"18F106A7", "Frame"="VCU07toFiveInOneRelay\ndatabase", "NameShort"="VCU07FiveInOneBrkResistRelayCmd", "StartBit"=11, "NumBits"=1, "Min"=0.0, "Max"=1.0, "ScaleFac"=1.0, "ScaleOff"=0.0}, {"18F106A7", "Frame"="VCU07toFiveInOneRelay\ndatabase", "NameShort"="VCU07FiveInOneDCDCRelayCmd", "StartBit"=5, "NumBits"=1, "Min"=0.0, "Max"=1.0, "ScaleFac"=1.0, "ScaleOff"=0.0}, {"18F106A7", "Frame"="VCU07toFiveInOneRelay\ndatabase", "NameShort"="VCU07FiveInOneDefrostRelayCmd", "StartBit"=1, "NumBits"=1, "Min"=0.0, "Max"=1.0, "ScaleFac"=1.0, "ScaleOff"=0.0}, {"18F106A7", "Frame"="VCU07toFiveInOneRelay\ndatabase", "NameShort"="VCU07FiveInOneEHPSRelayCmd", "StartBit"=4, "NumBits"=1, "Min"=0.0, "Max"=1.0, "ScaleFac"=1.0, "ScaleOff"=0.0}, {"18F106A7", "Frame"="VCU07toFiveInOneRelay\ndatabase", "NameShort"="VCU07FiveInOneHeatRelayCmd", "StartBit"=0, "NumBits"=1, "Min"=0.0, "Max"=1.0, "ScaleFac"=1.0, "ScaleOff"=0.0}, {"18F106A7", "Frame"="VCU07toFiveInOneRelay\ndatabase", "NameShort"="VCU07FiveInOneLife", "StartBit"=56, "NumBits"=8, "Min"=0.0, "Max"=255.0, "ScaleFac"=1.0, "ScaleOff"=0.0}, {"18F106A7", "Frame"="VCU07toFiveInOneRelay\ndatabase", "NameShort"="VCU07FiveInOneMtrRelayCmd", "StartBit"=6, "NumBits"=1, "Min"=0.0, "Max"=1.0, "ScaleFac"=1.0, "ScaleOff"=0.0}, {"18F106A7", "Frame"="VCU07toFiveInOneRelay\ndatabase", "NameShort"="VCU07FiveInOnePrechgRelayCmd", "StartBit"=7, "NumBits"=1, "Min"=0.0, "Max"=1.0, "ScaleFac"=1.0, "ScaleOff"=0.0}, {"18F108A7", "Frame"="VCU08toAirCompr1\ndatabase", "NameShort"="VCU08AirComprAssignRPM", "StartBit"=8, "NumBits"=16, "Min"=0.0, "Max"=5000.0, "ScaleFac"=0.125, "ScaleOff"=0.0}, {"18F108A7", "Frame"="VCU08toAirCompr1\ndatabase", "NameShort"="VCU08AirComprEnbl1", "StartBit"=0, "NumBits"=2, "Min"=0.0, "Max"=3.0, "ScaleFac"=1.0, "ScaleOff"=0.0}, {"18F108A7", "Frame"="VCU08toAirCompr1\ndatabase", "NameShort"="VCU08AirComprEnbl2", "StartBit"=2, "NumBits"=2, "Min"=0.0, "Max"=3.0, "ScaleFac"=1.0, "ScaleOff"=0.0}, {"18F108A7", "Frame"="VCU08toAirCompr1\ndatabase", "NameShort"="VCU08AirComprLife", "StartBit"=56, "NumBits"=8, "Min"=0.0, "Max"=255.0, "ScaleFac"=1.0, "ScaleOff"=0.0}, {"18F109A7", "Frame"="VCU09toAirCompr2\ndatabase", "NameShort"="VCU09AirComprAssignRPM", "StartBit"=8, "NumBits"=16, "Min"=0.0, "Max"=5000.0, "ScaleFac"=0.125, "ScaleOff"=0.0}, {"18F109A7", "Frame"="VCU09toAirCompr2\ndatabase", "NameShort"="VCU09AirComprEnbl1", "StartBit"=0, "NumBits"=2, "Min"=0.0, "Max"=3.0, "ScaleFac"=1.0, "ScaleOff"=0.0}, {"18F109A7", "Frame"="VCU09toAirCompr2\ndatabase", "NameShort"="VCU09AirComprEnbl2", "StartBit"=2, "NumBits"=2, "Min"=0.0, "Max"=3.0, "ScaleFac"=1.0, "ScaleOff"=0.0}, {"18F109A7", "Frame"="VCU09toAirCompr2\ndatabase", "NameShort"="VCU09AirComprLife", "StartBit"=56, "NumBits"=8, "Min"=0.0, "Max"=255.0, "ScaleFac"=1.0, "ScaleOff"=0.0}, {"CF109A7", "Frame"="VCU10toBrkResistNBMS\ndatabase", "NameShort"="VCU10BattMainRelayCmd", "StartBit"=55, "NumBits"=1, "Min"=0.0, "Max"=1.0, "ScaleFac"=1.0, "ScaleOff"=0.0}, {"CF109A7", "Frame"="VCU10toBrkResistNBMS\ndatabase", "NameShort"="VCU10BattMaxChgPowAllowed", "StartBit"=16, "NumBits"=16, "Min"=0.0, "Max"=500.0, "ScaleFac"=1.0, "ScaleOff"=0.0}, {"CF109A7", "Frame"="VCU10toBrkResistNBMS\ndatabase", "NameShort"="VCU10BrkResistNBMSLife", "StartBit"=56, "NumBits"=8, "Min"=0.0, "Max"=255.0, "ScaleFac"=1.0, "ScaleOff"=0.0}, {"CF109A7", "Frame"="VCU10toBrkResistNBMS\ndatabase", "NameShort"="VCU10BrkResistPowCmd", "StartBit"=47, "NumBits"=1, "Min"=0.0, "Max"=1.0, "ScaleFac"=1.0, "ScaleOff"=0.0}, {"CF109A7", "Frame"="VCU10toBrkResistNBMS\ndatabase", "NameShort"="VCU10BrkResistPowConsumpReq", "StartBit"=0, "NumBits"=16, "Min"=0.0, "Max"=500.0, "ScaleFac"=1.0, "ScaleOff"=0.0}, {"CF109A7", "Frame"="VCU10toBrkResistNBMS\ndatabase", "NameShort"="VCU10BrkResistorPowONOFFCmd", "StartBit"=46, "NumBits"=1, "Min"=0.0, "Max"=1.0, "ScaleFac"=1.0, "ScaleOff"=0.0}, {"18F10BA7", "Frame"="VCU11EVEff\ndatabase", "NameShort"="VCU11AvgPowConsump", "StartBit"=16, "NumBits"=16, "Min"=0.0, "Max"=5000.0, "ScaleFac"=0.1, "ScaleOff"=0.0}, {"18F10BA7", "Frame"="VCU11EVEff\ndatabase", "NameShort"="VCU11IPLife", "StartBit"=56, "NumBits"=8, "Min"=0.0, "Max"=255.0, "ScaleFac"=1.0, "ScaleOff"=0.0}, {"18F10BA7", "Frame"="VCU11EVEff\ndatabase", "NameShort"="VCU11InstantPowConsump", "StartBit"=0, "NumBits"=16, "Min"=0.0, "Max"=5000.0, "ScaleFac"=0.1, "ScaleOff"=0.0}, {"18F10BA7", "Frame"="VCU11EVEff\ndatabase", "NameShort"="VCU11RemainMileage", "StartBit"=32, "NumBits"=16, "Min"=0.0, "Max"=5000.0, "ScaleFac"=1.0, "ScaleOff"=0.0}, {"18FB01A7", "Frame"="VCU12AVAS\ndatabase", "NameShort"="VCU12AVASAcousticVehicleAlertSys", "StartBit"=12, "NumBits"=4, "Min"=0.0, "Max"=15.0, "ScaleFac"=1.0, "ScaleOff"=0.0}, {"18FEC1A7", "Frame"="VCU13Mileage\ndatabase", "NameShort"="VCU13MileageTotalOdometer", "StartBit"=0, "NumBits"=32, "Min"=0.0, "Max"=21055406.0, "ScaleFac"=0.005, "ScaleOff"=0.0}, {"18FEF117", "Frame"="VCU14CCVS\ndatabase", "NameShort"="VCU14CCVSBrkSwitch", "StartBit"=28, "NumBits"=2, "Min"=0.0, "Max"=3.0, "ScaleFac"=1.0, "ScaleOff"=0.0}, {"18FEF117", "Frame"="VCU14CCVS\ndatabase", "NameShort"="VCU14CCVSClutchSwitch", "StartBit"=30, "NumBits"=2, "Min"=0.0, "Max"=3.0, "ScaleFac"=1.0, "ScaleOff"=0.0}, {"18FEF117", "Frame"="VCU14CCVS\ndatabase", "NameShort"="VCU14CCVSCruiseCtrlAccSwitch", "StartBit"=38, "NumBits"=2, "Min"=0.0, "Max"=3.0, "ScaleFac"=1.0, "ScaleOff"=0.0}, {"18FEF117", "Frame"="VCU14CCVS\ndatabase", "NameShort"="VCU14CCVSCruiseCtrlActive", "StartBit"=24, "NumBits"=2, "Min"=0.0, "Max"=3.0, "ScaleFac"=1.0, "ScaleOff"=0.0}, {"18FEF117", "Frame"="VCU14CCVS\ndatabase", "NameShort"="VCU14CCVSCruiseCtrlCoastSwitch", "StartBit"=34, "NumBits"=2, "Min"=0.0, "Max"=3.0, "ScaleFac"=1.0, "ScaleOff"=0.0}, {"18FEF117", "Frame"="VCU14CCVS\ndatabase", "NameShort"="VCU14CCVSCruiseCtrlEnblSwitch", "StartBit"=26, "NumBits"=2, "Min"=0.0, "Max"=3.0, "ScaleFac"=1.0, "ScaleOff"=0.0}, {"18FEF117", "Frame"="VCU14CCVS\ndatabase", "NameShort"="VCU14CCVSCruiseCtrlPauseSwitch", "StartBit"=4, "NumBits"=2, "Min"=0.0, "Max"=3.0, "ScaleFac"=1.0, "ScaleOff"=0.0}, {"18FEF117", "Frame"="VCU14CCVS\ndatabase", "NameShort"="VCU14CCVSCruiseCtrlResumeSwitch", "StartBit"=36, "NumBits"=2, "Min"=0.0, "Max"=3.0, "ScaleFac"=1.0, "ScaleOff"=0.0}, {"18FEF117", "Frame"="VCU14CCVS\ndatabase", "NameShort"="VCU14CCVSCruiseCtrlSetSpeed", "StartBit"=40, "NumBits"=8, "Min"=0.0, "Max"=255.0, "ScaleFac"=1.0, "ScaleOff"=0.0}, {"18FEF117", "Frame"="VCU14CCVS\ndatabase", "NameShort"="VCU14CCVSCruiseCtrlSetSwitch", "StartBit"=32, "NumBits"=2, "Min"=0.0, "Max"=3.0, "ScaleFac"=1.0, "ScaleOff"=0.0}, {"18FEF117", "Frame"="VCU14CCVS\ndatabase", "NameShort"="VCU14CCVSCruiseCtrlState", "StartBit"=53, "NumBits"=3, "Min"=0.0, "Max"=7.0, "ScaleFac"=1.0, "ScaleOff"=0.0}, {"18FEF117", "Frame"="VCU14CCVS\ndatabase", "NameShort"="VCU14CCVSEngIdleDecrementSwitch", "StartBit"=58, "NumBits"=2, "Min"=0.0, "Max"=3.0, "ScaleFac"=1.0, "ScaleOff"=0.0}, {"18FEF117", "Frame"="VCU14CCVS\ndatabase", "NameShort"="VCU14CCVSEngIdleIncrementSwitch", "StartBit"=56, "NumBits"=2, "Min"=0.0, "Max"=3.0, "ScaleFac"=1.0, "ScaleOff"=0.0}, {"18FEF117", "Frame"="VCU14CCVS\ndatabase", "NameShort"="VCU14CCVSEngShutdownOvrSwitch", "StartBit"=62, "NumBits"=2, "Min"=0.0, "Max"=3.0, "ScaleFac"=1.0, "ScaleOff"=0.0}, {"18FEF117", "Frame"="VCU14CCVS\ndatabase", "NameShort"="VCU14CCVSEngTestModeSwitch", "StartBit"=60, "NumBits"=2, "Min"=0.0, "Max"=3.0, "ScaleFac"=1.0, "ScaleOff"=0.0}, {"18FEF117", "Frame"="VCU14CCVS\ndatabase", "NameShort"="VCU14CCVSPTOGovernorState", "StartBit"=48, "NumBits"=5, "Min"=0.0, "Max"=31.0, "ScaleFac"=1.0, "ScaleOff"=0.0}, {"18FEF117", "Frame"="VCU14CCVS\ndatabase", "NameShort"="VCU14CCVSParkBrkReleaseInhibitRq", "StartBit"=6, "NumBits"=2, "Min"=0.0, "Max"=3.0, "ScaleFac"=1.0, "ScaleOff"=0.0}, {"18FEF117", "Frame"="VCU14CCVS\ndatabase", "NameShort"="VCU14CCVSParkingBrkSwitch", "StartBit"=2, "NumBits"=2, "Min"=0.0, "Max"=3.0, "ScaleFac"=1.0, "ScaleOff"=0.0}, {"18FEF117", "Frame"="VCU14CCVS\ndatabase", "NameShort"="VCU14CCVSTwoSpeedAxleSwitch", "StartBit"=0, "NumBits"=2, "Min"=0.0, "Max"=3.0, "ScaleFac"=1.0, "ScaleOff"=0.0}, {"18FEF117", "Frame"="VCU14CCVS\ndatabase", "NameShort"="VCU14CCVSWheelBasedVehicleSpeed", "StartBit"=8, "NumBits"=16, "Min"=0.0, "Max"=250.996, "ScaleFac"=0.00390625, "ScaleOff"=0.0}, {"18F10CA7", "Frame"="VCU15VIN\ndatabase", "NameShort"="VCU15VINPkgNum", "StartBit"=0, "NumBits"=8, "Min"=0.0, "Max"=255.0, "ScaleFac"=1.0, "ScaleOff"=0.0}, {"18F10CA7", "Frame"="VCU15VIN\ndatabase", "NameShort"="VCU15VINcode0", "StartBit"=8, "NumBits"=8, "Min"=0.0, "Max"=255.0, "ScaleFac"=1.0, "ScaleOff"=0.0}, {"18F10CA7", "Frame"="VCU15VIN\ndatabase", "NameShort"="VCU15VINcode1", "StartBit"=16, "NumBits"=8, "Min"=0.0, "Max"=255.0, "ScaleFac"=1.0, "ScaleOff"=0.0}, {"18F10CA7", "Frame"="VCU15VIN\ndatabase", "NameShort"="VCU15VINcode2", "StartBit"=24, "NumBits"=8, "Min"=0.0, "Max"=255.0, "ScaleFac"=1.0, "ScaleOff"=0.0}, {"18F10CA7", "Frame"="VCU15VIN\ndatabase", "NameShort"="VCU15VINcode3", "StartBit"=32, "NumBits"=8, "Min"=0.0, "Max"=255.0, "ScaleFac"=1.0, "ScaleOff"=0.0}, {"18F10CA7", "Frame"="VCU15VIN\ndatabase", "NameShort"="VCU15VINcode4", "StartBit"=40, "NumBits"=8, "Min"=0.0, "Max"=255.0, "ScaleFac"=1.0, "ScaleOff"=0.0}, {"18F10CA7", "Frame"="VCU15VIN\ndatabase", "NameShort"="VCU15VINcode5", "StartBit"=48, "NumBits"=8, "Min"=0.0, "Max"=255.0, "ScaleFac"=1.0, "ScaleOff"=0.0}, {"18F10CA7", "Frame"="VCU15VIN\ndatabase", "NameShort"="VCU15VINcode6", "StartBit"=56, "NumBits"=8, "Min"=0.0, "Max"=255.0, "ScaleFac"=1.0, "ScaleOff"=0.0}, {"CF101D0", "Frame"="VCUtoINVT\ndatabase", "NameShort"="VCUtoINVTACHVPowReq", "StartBit"=24, "NumBits"=2, "Min"=0.0, "Max"=3.0, "ScaleFac"=1.0, "ScaleOff"=0.0}, {"CF101D0", "Frame"="VCUtoINVT\ndatabase", "NameShort"="VCUtoINVTLife", "StartBit"=56, "NumBits"=8, "Min"=0.0, "Max"=255.0, "ScaleFac"=1.0, "ScaleOff"=0.0}, {"CF101D0", "Frame"="VCUtoINVT\ndatabase", "NameShort"="VCUtoINVTMCUHVPowReq", "StartBit"=8, "NumBits"=2, "Min"=0.0, "Max"=3.0, "ScaleFac"=1.0, "ScaleOff"=0.0}, {"CF103D0", "Frame"="VCUtoINVT2\ndatabase", "NameShort"="VCUtoINVT2DCDCEnbl", "StartBit"=4, "NumBits"=2, "Min"=0.0, "Max"=1.0, "ScaleFac"=1.0, "ScaleOff"=0.0}, {"CF103D0", "Frame"="VCUtoINVT2\ndatabase", "NameShort"="VCUtoINVT2DCDCOUTVolt", "StartBit"=8, "NumBits"=16, "Min"=0.0, "Max"=6553.5, "ScaleFac"=0.1, "ScaleOff"=0.0}, {"CF103D0", "Frame"="VCUtoINVT2\ndatabase", "NameShort"="VCUtoINVT2EACEnbl", "StartBit"=2, "NumBits"=2, "Min"=0.0, "Max"=1.0, "ScaleFac"=1.0, "ScaleOff"=0.0}, {"CF103D0", "Frame"="VCUtoINVT2\ndatabase", "NameShort"="VCUtoINVT2EACmode", "StartBit"=7, "NumBits"=1, "Min"=0.0, "Max"=1.0, "ScaleFac"=1.0, "ScaleOff"=0.0}, {"CF103D0", "Frame"="VCUtoINVT2\ndatabase", "NameShort"="VCUtoINVT2EACrpm", "StartBit"=40, "NumBits"=16, "Min"=-5000.0, "Max"=5000.0, "ScaleFac"=0.5, "ScaleOff"=-5000.0}, {"CF103D0", "Frame"="VCUtoINVT2\ndatabase", "NameShort"="VCUtoINVT2EHPSEnbl", "StartBit"=0, "NumBits"=2, "Min"=0.0, "Max"=1.0, "ScaleFac"=1.0, "ScaleOff"=0.0}, {"CF103D0", "Frame"="VCUtoINVT2\ndatabase", "NameShort"="VCUtoINVT2EHPSmode", "StartBit"=6, "NumBits"=1, "Min"=0.0, "Max"=1.0, "ScaleFac"=1.0, "ScaleOff"=0.0}, {"CF103D0", "Frame"="VCUtoINVT2\ndatabase", "NameShort"="VCUtoINVT2EHPSrpm", "StartBit"=24, "NumBits"=16, "Min"=-5000.0, "Max"=5000.0, "ScaleFac"=0.5, "ScaleOff"=-5000.0}, {"CF103D0", "Frame"="VCUtoINVT2\ndatabase", "NameShort"="VCUtoINVT2Life", "StartBit"=56, "NumBits"=8, "Min"=0.0, "Max"=255.0, "ScaleFac"=1.0, "ScaleOff"=0.0}]
  in  "error in (no error)":errorcluster
  out "error out":errorcluster
  # "Configure"
  # "Send Message"
  # "Received Messages"
  # "Time Stamp   Message Id  Flags  DLC     Data"
  # "8"
  # "16"
  # "24"
  # "32"
  # "40"
  # "48"
  # "車身:250K\n動力:500K"
  # "56"
  # "64"
  # "VCU1:ID=0x0CF101A7"
